vi "NewChicagoStyleClamPizza.vi"(8 "error in (no error)":errorcluster) -> (0 "error out":errorcluster, 3 "ChicagoStyleClamPizza":refnum<class "ChicagoStyleClamPizza.lvclass">)   [LabVIEW 2020, in "FactoryMethod.lvlib" / "PizzaFactoryMethod.lvlib" / "ChicagoStyleClamPizza.lvclass"]
uses:
  ChicagoStyleClamPizza.lvclass
  ChicagoStyleClamPizza.lvclass/ChicagoStyleClamPizza.ctl
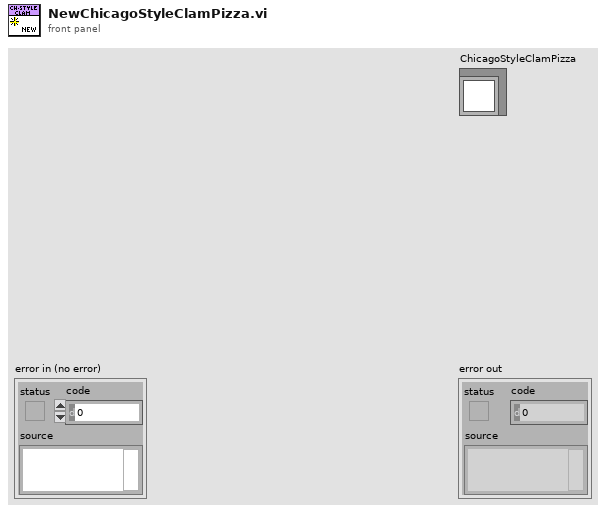
[diagram p1: front panel]
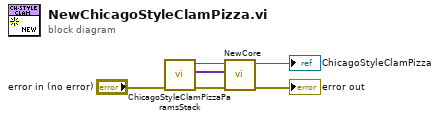
[diagram p0: block diagram]
diagram:
  n1 = call "ChicagoStyleClamPizzaParamsStack.vi"("error iN"="error in (no error)") -> ("error out"=w6:errorcluster, "HierarchyParams"=w5:variant[], "ChicagoStyleClamPizza"=w1:refnum<class "ChicagoStyleClamPizza.lvclass">)  [unwired: 8 in]
  n2 = call-dynamic "NewCore.vi"("error in (no error)"=w6, "ParamsArray"=w5, "ChicagoStyleClamPizza"=w1) -> ("error out"=→"error out":errorcluster, "ChicagoStyleClamPizza"=→"ChicagoStyleClamPizza":refnum<class "ChicagoStyleClamPizza.lvclass">)  [unwired: 7 in]
